vi "SetPosition.vi"(7 "AltPipe?":bool, 8 "error in (no error)":errorcluster, 9 "Position":T1=enum."C0, Cargo Ground", 10 "Hach Grabed?":bool, 11 "Elevator Concrete in":refnum<class "Elevator Arm.lvclass">) -> (0 "error out":errorcluster, 3 "Elevator Concrete out":refnum<class "Elevator Arm.lvclass">)   [LabVIEW 2018, in "Elevator.lvlib" / "Elevator Arm.lvclass"]
uses:
  Elevator Arm.lvclass
  C:/Users/Howdy Bots/Documents/2019DeepSpace/Classes/Elevator/Elevator.lvclass
  Controls/Elevator Position.ctl
  Elevator Arm.lvclass/Elevator Arm.ctl
  Elevator.lvclass/Elevator.ctl
  Public Methods/Read Arm Position Values.vi
  <vilib>/Rock Robotics/Network Tables/NT Write Number.vi
  <vilib>/Rock Robotics/Network Tables/NT Write String.vi
  Elevator.lvclass
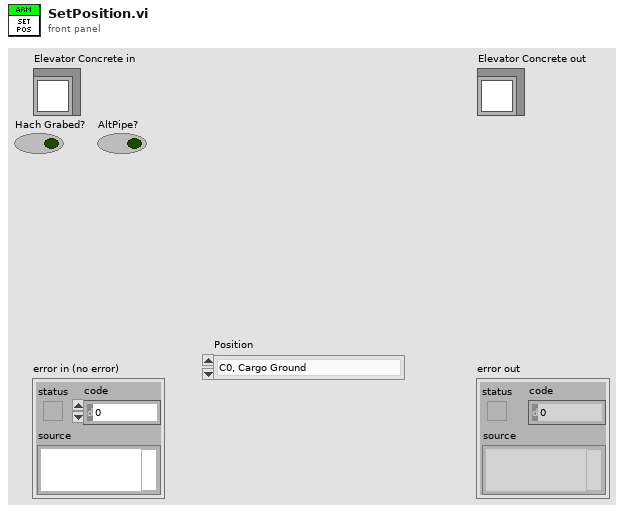
[diagram p1: front panel]
types:
  T1 = typedef "Elevator.lvlib/Elevator.lvclass/Elevator Position.ctl" = enum16{"CS, Cargo Ship Cargo", "C0, Cargo Ground", "C1, LV1 Cargo", "C2, LV2 Cargo", "C3, LV3 Cargo", "H0, LV1 Hatch", "H1, LV2 Hatch", "H2, LV3 Hatch"}
  T2 = typedef "Elevator.lvlib/Elevator.lvclass/Arm Position Values.ctl" = cluster{"C0 Arm":dbl, "C1 Arm":dbl, "C2 Arm":dbl, "H1 Arm":dbl, "H2 Arm":dbl, "C0 Wrist":dbl, "C1 Wrist ":dbl, "C2 Wrist":dbl, "H1 Wrist":dbl, "H2 Wrist":dbl, "Deploy Arm":dbl, "Deploy Wrist":dbl, "Climb Arm":dbl, "Climb Wrist":dbl, "Stowed Arm":dbl, "Stowed Wrist":dbl, "CS":dbl, "C0":dbl, "C1":dbl, "C2":dbl, "C3":dbl, "H0":dbl, "H1":dbl, "H2":dbl}
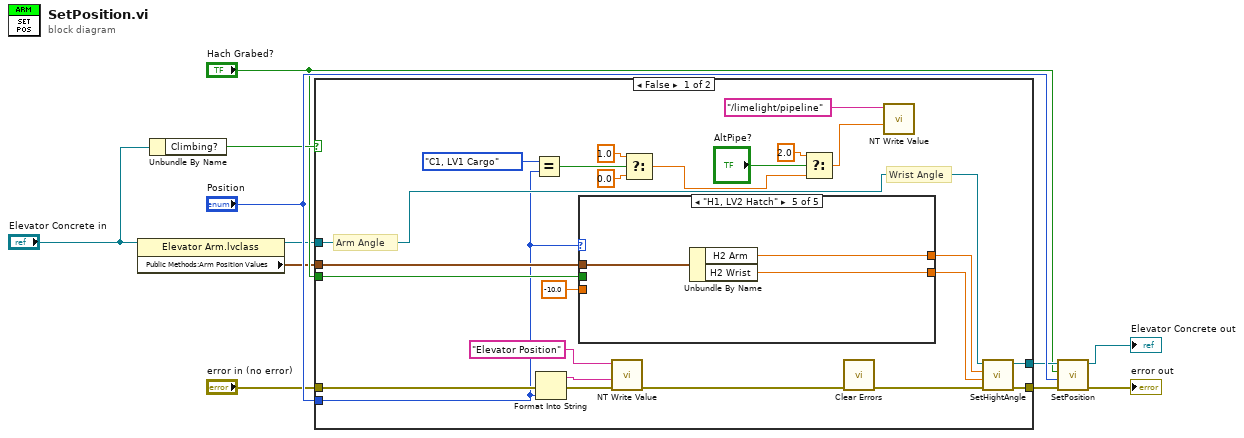
[diagram p0: block diagram]
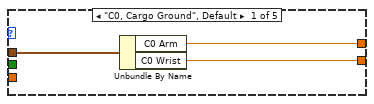
[diagram p2: hidden frame]
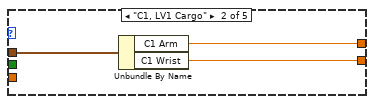
[diagram p3: hidden frame]
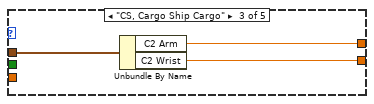
[diagram p4: hidden frame]
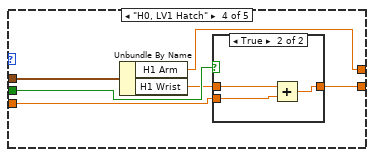
[diagram p5: hidden frame]
diagram:
  n1 = property class="Elevator Arm.lvclass"(reference="Elevator Concrete in") -> (reference out=w2:refnum<class "Elevator Arm.lvclass">, "Public Methods:Arm Position Values"=w1:T2)  [unwired: 1 in, 1 out]
  n2 = Unbundle By Name("Elevator Concrete in") -> ("Climbing?"=w4:bool)
  n3 = case shown="False" w4 {
    tunnel: "Position" -> [w17 _]
    tunnel: "error in (no error)" -> [w24 w58]
    tunnel: w2 -> [w33 w59]
    tunnel: [w31 w58] -> w6
    tunnel: [w32 w59] -> w5
    tunnel: "Hach Grabed?" -> [w29 _]
    tunnel: w1 -> [w28 _]
    frame False {
      # "Wrist Angle"
      # "Arm Angle"
      n4 = Equal?(x=Elevator_Position."C1, LV1 Cargo" ("Position"), y=w17) -> (x = y?=w21:bool)
      n5 = Format Into String(error in=w24, w17) -> (resulting string=w22:string, error out=w25:errorcluster)  [unwired: 2 in]
      n6 = case shown="\"H1, LV2 Hatch\"" w17 {
        tunnel: [w36 w39 w42 w48 w55] -> w34
        tunnel: [w37 w40 w43 w46 w56] -> w35
        tunnel: -10.0 -> [_ _ _ w49 _]
        tunnel: w29 -> [_ _ _ w50 _]
        tunnel: w28 -> [w38 w41 w44 w47 w57]
        frame "C0, Cargo Ground", Default {
          n7 = Unbundle By Name(w38) -> ("C0 Arm"=w37:dbl, "C0 Wrist"=w36:dbl)
        }
        frame "C1, LV1 Cargo" {
          n8 = Unbundle By Name(w41) -> ("C1 Arm"=w40:dbl, "C1 Wrist"=w39:dbl)
        }
        frame "CS, Cargo Ship Cargo" {
          n9 = Unbundle By Name(w44) -> ("C2 Arm"=w43:dbl, "C2 Wrist"=w42:dbl)
        }
        frame "H0, LV1 Hatch" {
          n10 = Unbundle By Name(w47) -> ("H1 Arm"=w46:dbl, "H1 Wrist"=w45:dbl)
          n11 = case shown="True" w50 {
            tunnel: [w51 w52] -> w48
            tunnel: w45 -> [w51 w54]
            tunnel: w49 -> [_ w53]
            frame False {
            }
            frame True {
              n12 = Add(x=w54, y=w53) -> (x+y=w52:dbl)
            }
          }
        }
        frame "H1, LV2 Hatch" {
          n13 = Unbundle By Name(w57) -> ("H2 Arm"=w56:dbl, "H2 Wrist"=w55:dbl)
        }
      }
      n14 = call-poly <vilib>:"NT Write Value.vi"("error in"=w25, "String"=w22, "Name"="Elevator Position") -> ("error out"=w27:errorcluster)  [unwired: 8 in]
      n15 = Select(t=1.0, s=w21, f=0.0) -> (s? t:f=w15:dbl)
      n16 = Select(t=2.0, s="AltPipe?", f=w15) -> (s? t:f=w14:dbl)
      n17 = call <vilib>:"Clear Errors.vi"("error in (no error)"=w27) -> ("error out"=w23:errorcluster)  [unwired: 5 in, 1 out]
      n18 = call-poly <vilib>:"NT Write Value.vi"("Numeric"=w14, "Name"="/limelight/pipeline") -> ()  [unwired: 9 in, 1 out]
      n19 = call-dynamic "SetHightAngle.vi"("error in (no error)"=w23, "Wrist (degrees)"=w34, "Main arm(degrees)"=w35, "Elevator Concrete in"=w33) -> ("error out"=w31:errorcluster, "Elevator Concrete out"=w32:refnum<class "Elevator Arm.lvclass">)  [unwired: 6 in]
    }
    frame True {
    }
  }
  n20 = call-parent "SetPosition.vi"("error in (no error)"=w6, "Position"="Position", "Hatch Grabbed?"="Hach Grabed?", "Elevator in"=w5) -> ("error out"=→"error out":errorcluster, "Elevator out"=→"Elevator Concrete out":refnum<class "Elevator Arm.lvclass">)  [unwired: 6 in]
